vi "Too Close to Starting WP.vi"() -> (0 "Too Close?":bool, 1 "Bearing to Avoid":dbl)   [LabVIEW 2009]
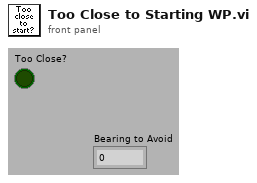
[diagram p1: front panel]
types:
  T1 = typedef "GPS Data.ctl" = cluster{"Latitude":dbl, "Longitude":dbl}
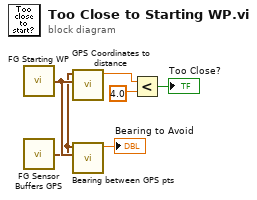
[diagram p0: block diagram]
diagram:
  n1 = call "FG Starting WP.vi"() -> ("Starting WP out"=w4:T1)  [unwired: 2 in]
  n2 = call "FG Sensor Buffers GPS.vi"() -> ("GPS Buffer out"=w2:T1)  [unwired: 2 in]
  n3 = call "GPS Coordinates to distance.vi"("GPS Co-ordinate 2"=w4, "GPS Co-ordinate 1"=w2) -> ("Distance"=w1:dbl)  [unwired: 9 in]
  n4 = call "Bearing between GPS pts.vi"("Pt.2"=w4, "Pt.1"=w2) -> ("Bearing Pt.1 to Pt.2"=→"Bearing to Avoid":dbl)  [unwired: 9 in]
  n5 = Less?(x=w1, y=4.0) -> (x < y?=→"Too Close?":bool)
